vi "Martinas Aging Program v1.0a.vi"() -> ()   [LabVIEW 2011]
uses:
  SubVIs/Control 3.ctl
panel:
  in  "Scan Switch":T1=TRUE
  out "TIMER":dbl format="%<%H:%M:%S>t"
  in  "Delete from Menu Ring":bool
  in  "User Set?":bool
  out "Show me Scan \nSettings JV set":T2={"Light Intensity (Suns)"=1.0, "Stabilization Time (s)"=5.0, "Maximum Voltage (V)"=0.0, "Minimum Voltage (V)"=-1.0, "Range Options"=0, "Scan Direction\nDU (T), UD (F)"=TRUE, "Step Size (V)"=0.01, "Source Delay (s)"=0.15} {"Range Options" items=["Auto Range", "Semi-Auto Range", "100 uA", "1 mA", "10 mA", "100 mA", "1A"]}
  in  "Add to Menu ring":bool
  in  "Scan Setting Name":string
  in  "Scan Settings JV":T2={"Light Intensity (Suns)"=1.0, "Stabilization Time (s)"=5.0, "Maximum Voltage (V)"=0.0, "Minimum Voltage (V)"=-1.0, "Range Options"=0, "Scan Direction\nDU (T), UD (F)"=TRUE, "Step Size (V)"=0.01, "Source Delay (s)"=0.15} {"Range Options" items=["Auto Range", "Semi-Auto Range", "100 uA", "1 mA", "10 mA", "100 mA", "1A"]}
  in  "Scan settings":u16(ring) items=["Regular", "Inverted"]
  out "JV Curve":cluster{"Y":dbl[], "Y":dbl[]}[](graph)
  out "Table":string[][](table)
  in  "Logout":bool
  in  "Login":bool
  out "Username":string caption="Logged in as:"
  in  "Sort by":u16(ring) items=["Cell position", "Cell label", "Time in rig"]
  in  "Sort Queue":bool
  in  "Upload to the Queue":bool
  in  "Queue":T3(array[cluster])=[{"Measure?"=TRUE, "Area (cm^2)"=0.0, "Cell Label"="", "Cell Description"="", "Cell Position"=0, "Time in rig (h)"=0.0, "Time to next scan (min)"=0.0, "Scan number"=0.0, "When did you stick it in?"=0.0, "Time between scans (min)"=0.0, "Time of the last scan(min)"=0.0, "Scan settings in queue"=0}, {"Measure?"=TRUE, "Area (cm^2)"=0.0, "Cell Label"="", "Cell Description"="", "Cell Position"=0, "Time in rig (h)"=0.0, "Time to next scan (min)"=0.0, "Scan number"=0.0, "When did you stick it in?"=0.0, "Time between scans (min)"=0.0, "Time of the last scan(min)"=0.0, "Scan settings in queue"=0}, {"Measure?"=TRUE, "Area (cm^2)"=0.0, "Cell Label"="", "Cell Description"="", "Cell Position"=0, "Time in rig (h)"=0.0, "Time to next scan (min)"=0.0, "Scan number"=0.0, "When did you stick it in?"=0.0, "Time between scans (min)"=0.0, "Time of the last scan(min)"=0.0, "Scan settings in queue"=0}, {"Measure?"=TRUE, "Area (cm^2)"=0.0, "Cell Label"="", "Cell Description"="", "Cell Position"=0, "Time in rig (h)"=0.0, "Time to next scan (min)"=0.0, "Scan number"=0.0, "When did you stick it in?"=0.0, "Time between scans (min)"=0.0, "Time of the last scan(min)"=0.0, "Scan settings in queue"=0}, {"Measure?"=TRUE, "Area (cm^2)"=0.0, "Cell Label"="", "Cell Description"="", "Cell Position"=0, "Time in rig (h)"=0.0, "Time to next scan (min)"=0.0, "Scan number"=0.0, "When did you stick it in?"=0.0, "Time between scans (min)"=0.0, "Time of the last scan(min)"=0.0, "Scan settings in queue"=0}, {"Measure?"=TRUE, "Area (cm^2)"=0.0, "Cell Label"="", "Cell Description"="", "Cell Position"=0, "Time in rig (h)"=0.0, "Time to next scan (min)"=0.0, "Scan number"=0.0, "When did you stick it in?"=0.0, "Time between scans (min)"=0.0, "Time of the last scan(min)"=0.0, "Scan settings in queue"=0}, {"Measure?"=TRUE, "Area (cm^2)"=0.0, "Cell Label"="", "Cell Description"="", "Cell Position"=0, "Time in rig (h)"=0.0, "Time to next scan (min)"=0.0, "Scan number"=0.0, "When did you stick it in?"=0.0, "Time between scans (min)"=0.0, "Time of the last scan(min)"=0.0, "Scan settings in queue"=0}, {"Measure?"=TRUE, "Area (cm^2)"=0.0, "Cell Label"="", "Cell Description"="", "Cell Position"=0, "Time in rig (h)"=0.0, "Time to next scan (min)"=0.0, "Scan number"=0.0, "When did you stick it in?"=0.0, "Time between scans (min)"=0.0, "Time of the last scan(min)"=0.0, "Scan settings in queue"=0}, {"Measure?"=TRUE, "Area (cm^2)"=0.0, "Cell Label"="", "Cell Description"="", "Cell Position"=0, "Time in rig (h)"=0.0, "Time to next scan (min)"=0.0, "Scan number"=0.0, "When did you stick it in?"=0.0, "Time between scans (min)"=0.0, "Time of the last scan(min)"=0.0, "Scan settings in queue"=0}, {"Measure?"=TRUE, "Area (cm^2)"=0.0, "Cell Label"="", "Cell Description"="", "Cell Position"=0, "Time in rig (h)"=0.0, "Time to next scan (min)"=0.0, "Scan number"=0.0, "When did you stick it in?"=0.0, "Time between scans (min)"=0.0, "Time of the last scan(min)"=0.0, "Scan settings in queue"=0}, {"Measure?"=TRUE, "Area (cm^2)"=0.0, "Cell Label"="", "Cell Description"="", "Cell Position"=0, "Time in rig (h)"=0.0, "Time to next scan (min)"=0.0, "Scan number"=0.0, "When did you stick it in?"=0.0, "Time between scans (min)"=0.0, "Time of the last scan(min)"=0.0, "Scan settings in queue"=0}, {"Measure?"=TRUE, "Area (cm^2)"=0.0, "Cell Label"="", "Cell Description"="", "Cell Position"=0, "Time in rig (h)"=0.0, "Time to next scan (min)"=0.0, "Scan number"=0.0, "When did you stick it in?"=0.0, "Time between scans (min)"=0.0, "Time of the last scan(min)"=0.0, "Scan settings in queue"=0}, {"Measure?"=TRUE, "Area (cm^2)"=0.0, "Cell Label"="", "Cell Description"="", "Cell Position"=0, "Time in rig (h)"=0.0, "Time to next scan (min)"=0.0, "Scan number"=0.0, "When did you stick it in?"=0.0, "Time between scans (min)"=0.0, "Time of the last scan(min)"=0.0, "Scan settings in queue"=0}, {"Measure?"=TRUE, "Area (cm^2)"=0.0, "Cell Label"="", "Cell Description"="", "Cell Position"=0, "Time in rig (h)"=0.0, "Time to next scan (min)"=0.0, "Scan number"=0.0, "When did you stick it in?"=0.0, "Time between scans (min)"=0.0, "Time of the last scan(min)"=0.0, "Scan settings in queue"=0}, {"Measure?"=TRUE, "Area (cm^2)"=0.0, "Cell Label"="", "Cell Description"="", "Cell Position"=0, "Time in rig (h)"=0.0, "Time to next scan (min)"=0.0, "Scan number"=0.0, "When did you stick it in?"=0.0, "Time between scans (min)"=0.0, "Time of the last scan(min)"=0.0, "Scan settings in queue"=0}, {"Measure?"=TRUE, "Area (cm^2)"=0.0, "Cell Label"="", "Cell Description"="", "Cell Position"=0, "Time in rig (h)"=0.0, "Time to next scan (min)"=0.0, "Scan number"=0.0, "When did you stick it in?"=0.0, "Time between scans (min)"=0.0, "Time of the last scan(min)"=0.0, "Scan settings in queue"=0}] {"Scan settings in queue" items=["Regular", "Inverted"]; "Time of the last scan(min)" format="%<%H:%M:%S>t"; "When did you stick it in?" format="%<%H:%M:%S>t"; "Time to next scan (min)" format="%<%H:%M:%S>t"; "Time in rig (h)" format="%<%H:%M:%S>t"}
  in  "Save Spreadsheet Path":path
  in  "Save to Spreadsheet?":bool
  in  "Upload Spreadsheet path":path
  in  "Upload from Spreadsheet?":bool
  in  "stop":bool
  in  "Cell Settings Array":T4(array[cluster])=[{"Measure?"=TRUE, "Area (cm^2)"=0.0, "Cell Label"="", "Cell Description"="", "Time between scans (min)"=0.0, "Cell Position"=0, "Scan settings in queue"=0}, {"Measure?"=TRUE, "Area (cm^2)"=0.0, "Cell Label"="", "Cell Description"="", "Time between scans (min)"=0.0, "Cell Position"=0, "Scan settings in queue"=0}, {"Measure?"=TRUE, "Area (cm^2)"=0.0, "Cell Label"="", "Cell Description"="", "Time between scans (min)"=0.0, "Cell Position"=0, "Scan settings in queue"=0}, {"Measure?"=TRUE, "Area (cm^2)"=0.0, "Cell Label"="", "Cell Description"="", "Time between scans (min)"=0.0, "Cell Position"=0, "Scan settings in queue"=0}, {"Measure?"=TRUE, "Area (cm^2)"=0.0, "Cell Label"="", "Cell Description"="", "Time between scans (min)"=0.0, "Cell Position"=0, "Scan settings in queue"=0}, {"Measure?"=TRUE, "Area (cm^2)"=0.0, "Cell Label"="", "Cell Description"="", "Time between scans (min)"=0.0, "Cell Position"=0, "Scan settings in queue"=0}, {"Measure?"=TRUE, "Area (cm^2)"=0.0, "Cell Label"="", "Cell Description"="", "Time between scans (min)"=0.0, "Cell Position"=0, "Scan settings in queue"=0}, {"Measure?"=TRUE, "Area (cm^2)"=0.0, "Cell Label"="", "Cell Description"="", "Time between scans (min)"=0.0, "Cell Position"=0, "Scan settings in queue"=0}, {"Measure?"=TRUE, "Area (cm^2)"=0.0, "Cell Label"="", "Cell Description"="", "Time between scans (min)"=0.0, "Cell Position"=0, "Scan settings in queue"=0}, {"Measure?"=TRUE, "Area (cm^2)"=0.0, "Cell Label"="", "Cell Description"="", "Time between scans (min)"=0.0, "Cell Position"=0, "Scan settings in queue"=0}, {"Measure?"=TRUE, "Area (cm^2)"=0.0, "Cell Label"="", "Cell Description"="", "Time between scans (min)"=0.0, "Cell Position"=0, "Scan settings in queue"=0}, {"Measure?"=TRUE, "Area (cm^2)"=0.0, "Cell Label"="", "Cell Description"="", "Time between scans (min)"=0.0, "Cell Position"=0, "Scan settings in queue"=0}, {"Measure?"=TRUE, "Area (cm^2)"=0.0, "Cell Label"="", "Cell Description"="", "Time between scans (min)"=0.0, "Cell Position"=0, "Scan settings in queue"=0}, {"Measure?"=TRUE, "Area (cm^2)"=0.0, "Cell Label"="", "Cell Description"="", "Time between scans (min)"=0.0, "Cell Position"=0, "Scan settings in queue"=0}, {"Measure?"=TRUE, "Area (cm^2)"=0.0, "Cell Label"="", "Cell Description"="", "Time between scans (min)"=0.0, "Cell Position"=0, "Scan settings in queue"=0}, {"Measure?"=TRUE, "Area (cm^2)"=0.0, "Cell Label"="", "Cell Description"="", "Time between scans (min)"=0.0, "Cell Position"=0, "Scan settings in queue"=0}] {"Scan settings in queue" items=["Regular", "Inverted"]}
  # "Time between Scans (min)"
  # "On = working cell\nOff = not working cell"
  # "Area"
  # "Label"
  # "Comment"
  # "Cell position"
  # "Scan Settings"
  # "Time between Scans (min)"
  # "Time since the last scan (min)"
  # "Scan\nnumber"
  # "When did you stick it in?"
  # "Time of the last scan"
  # "On = working cell\nOff = not working cell"
  # "Area"
  # "Label"
  # "Comment"
  # "Cell position"
  # "Time in rig"
  # "Scan Settings"
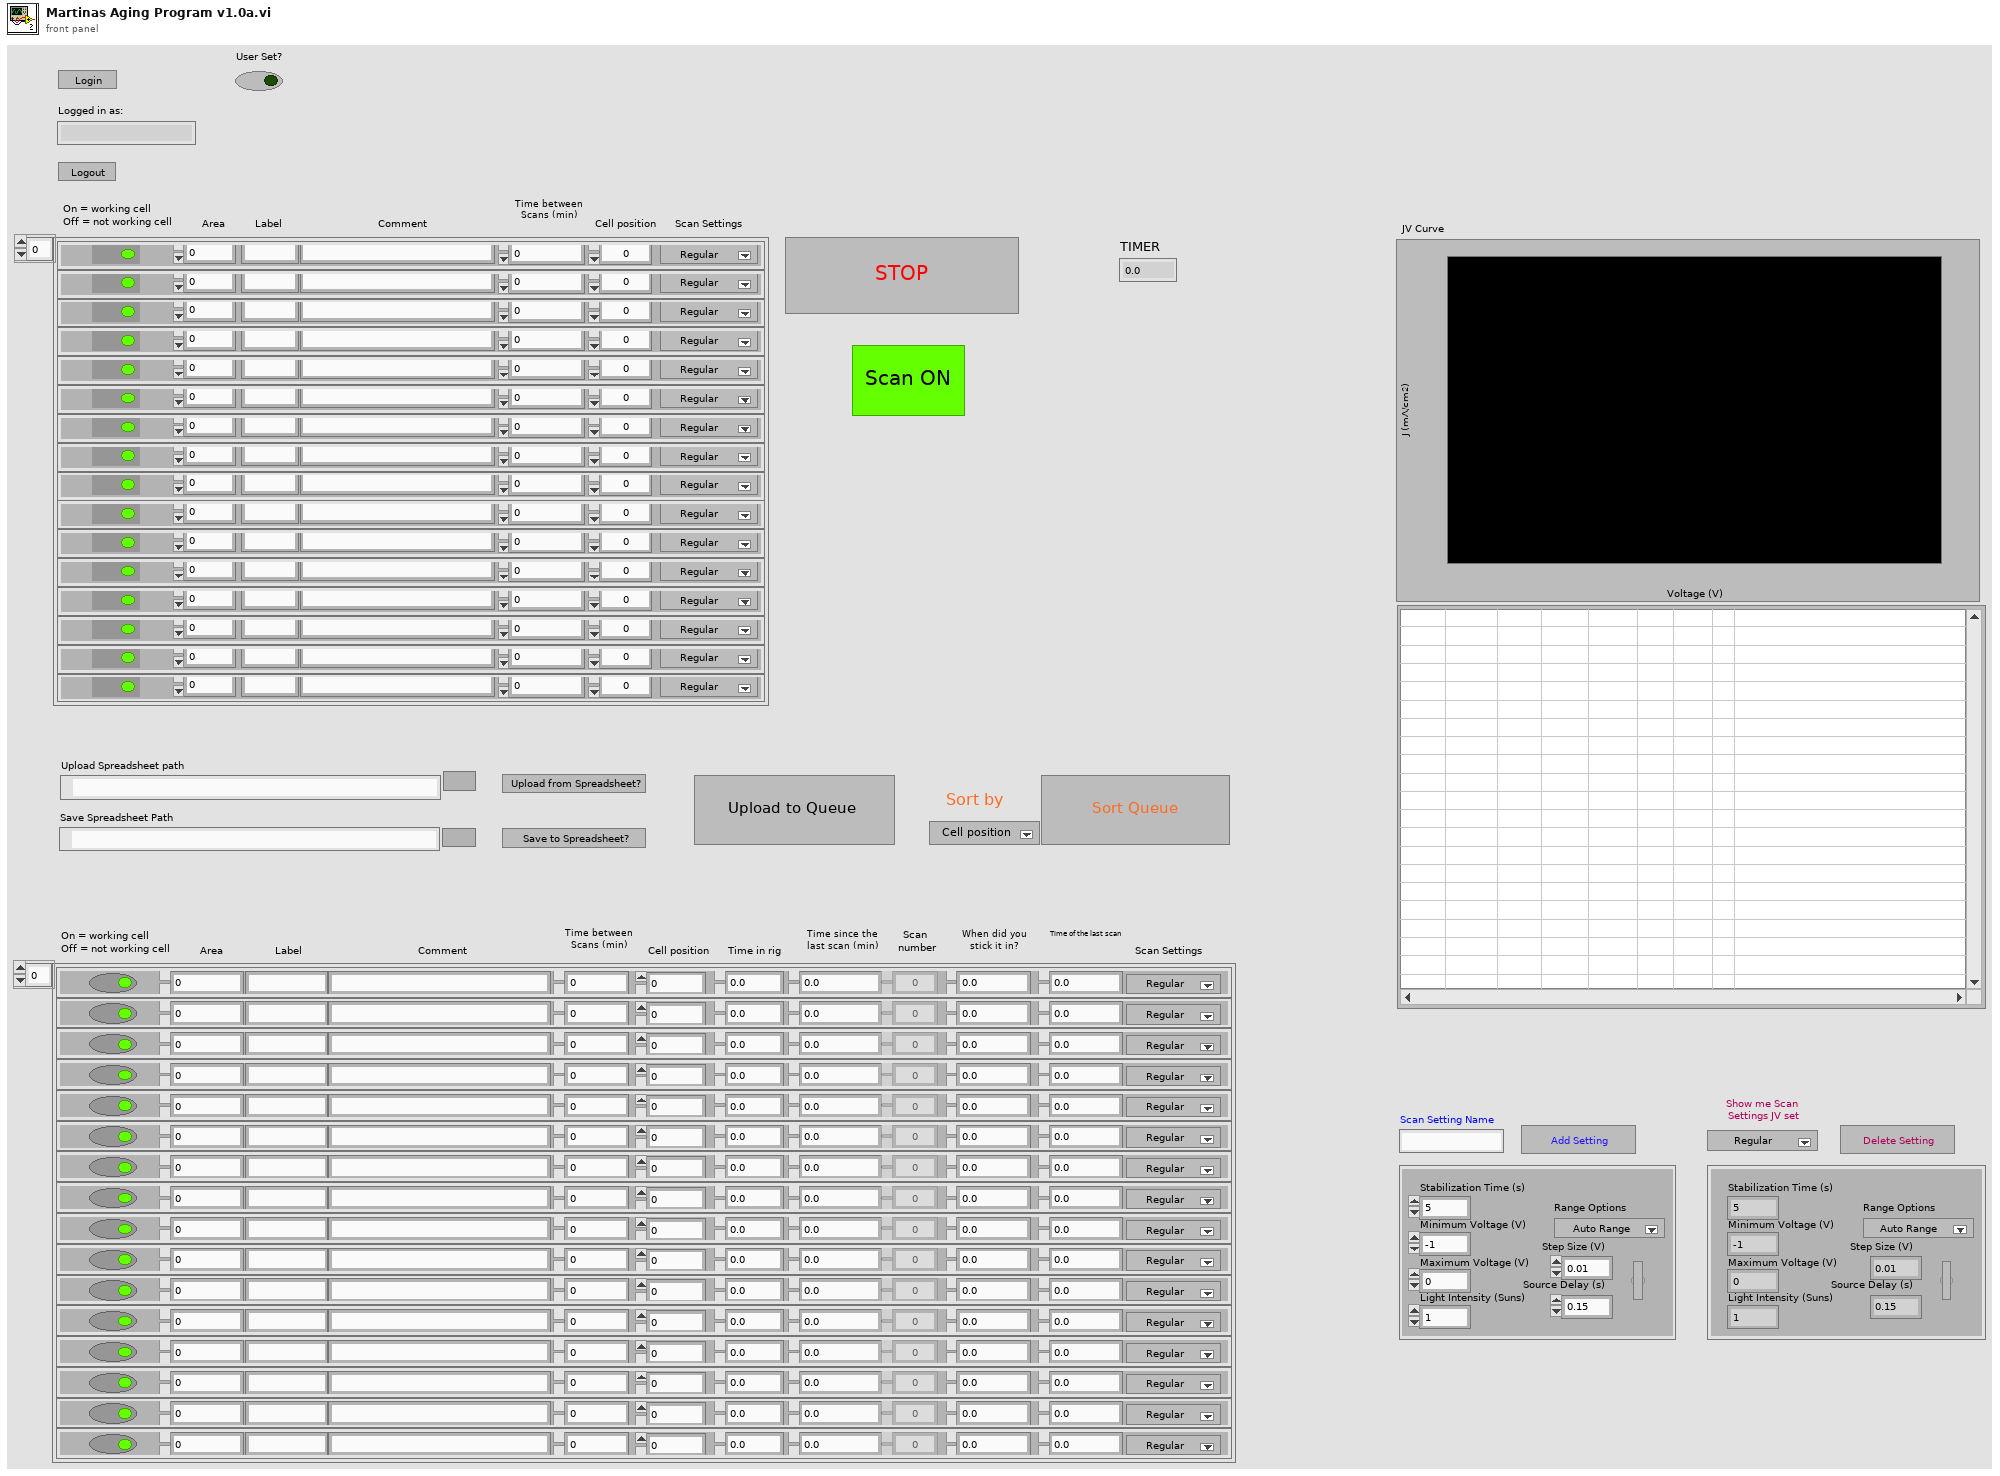
[diagram p1: front panel]
types:
  T1 = typedef "Control 3.ctl" = bool
  T2 = cluster{"Light Intensity (Suns)":dbl, "Stabilization Time (s)":dbl, "Maximum Voltage (V)":dbl, "Minimum Voltage (V)":dbl, "Range Options":u16, "Scan Direction\nDU (T), UD (F)":bool, "Step Size (V)":dbl, "Source Delay (s)":dbl}
  T3 = cluster{"Measure?":bool, "Area (cm^2)":dbl, "Cell Label":string, "Cell Description":string, "Cell Position":i32, "Time in rig (h)":dbl, "Time to next scan (min)":dbl, "Scan number":dbl, "When did you stick it in?":dbl, "Time between scans (min)":dbl, "Time of the last scan(min)":dbl, "Scan settings in queue":u16}[]
  T4 = cluster{"Measure?":bool, "Area (cm^2)":dbl, "Cell Label":string, "Cell Description":string, "Time between scans (min)":dbl, "Cell Position":i32, "Scan settings in queue":u16}[]
  T5 = cluster{"Light Intensity (Suns)":dbl, "Stabilization Time (s)":dbl, "Maximum Voltage (V)":dbl, "Minimum Voltage (V)":dbl, "Range Options":u16, "Scan Direction\nDU (T), UD (F)":bool, "Step Size (V)":dbl, "Source Delay (s)":dbl}[]
  T6 = enum8{"Enabled", "Disabled", "Disabled and Grayed Out"}
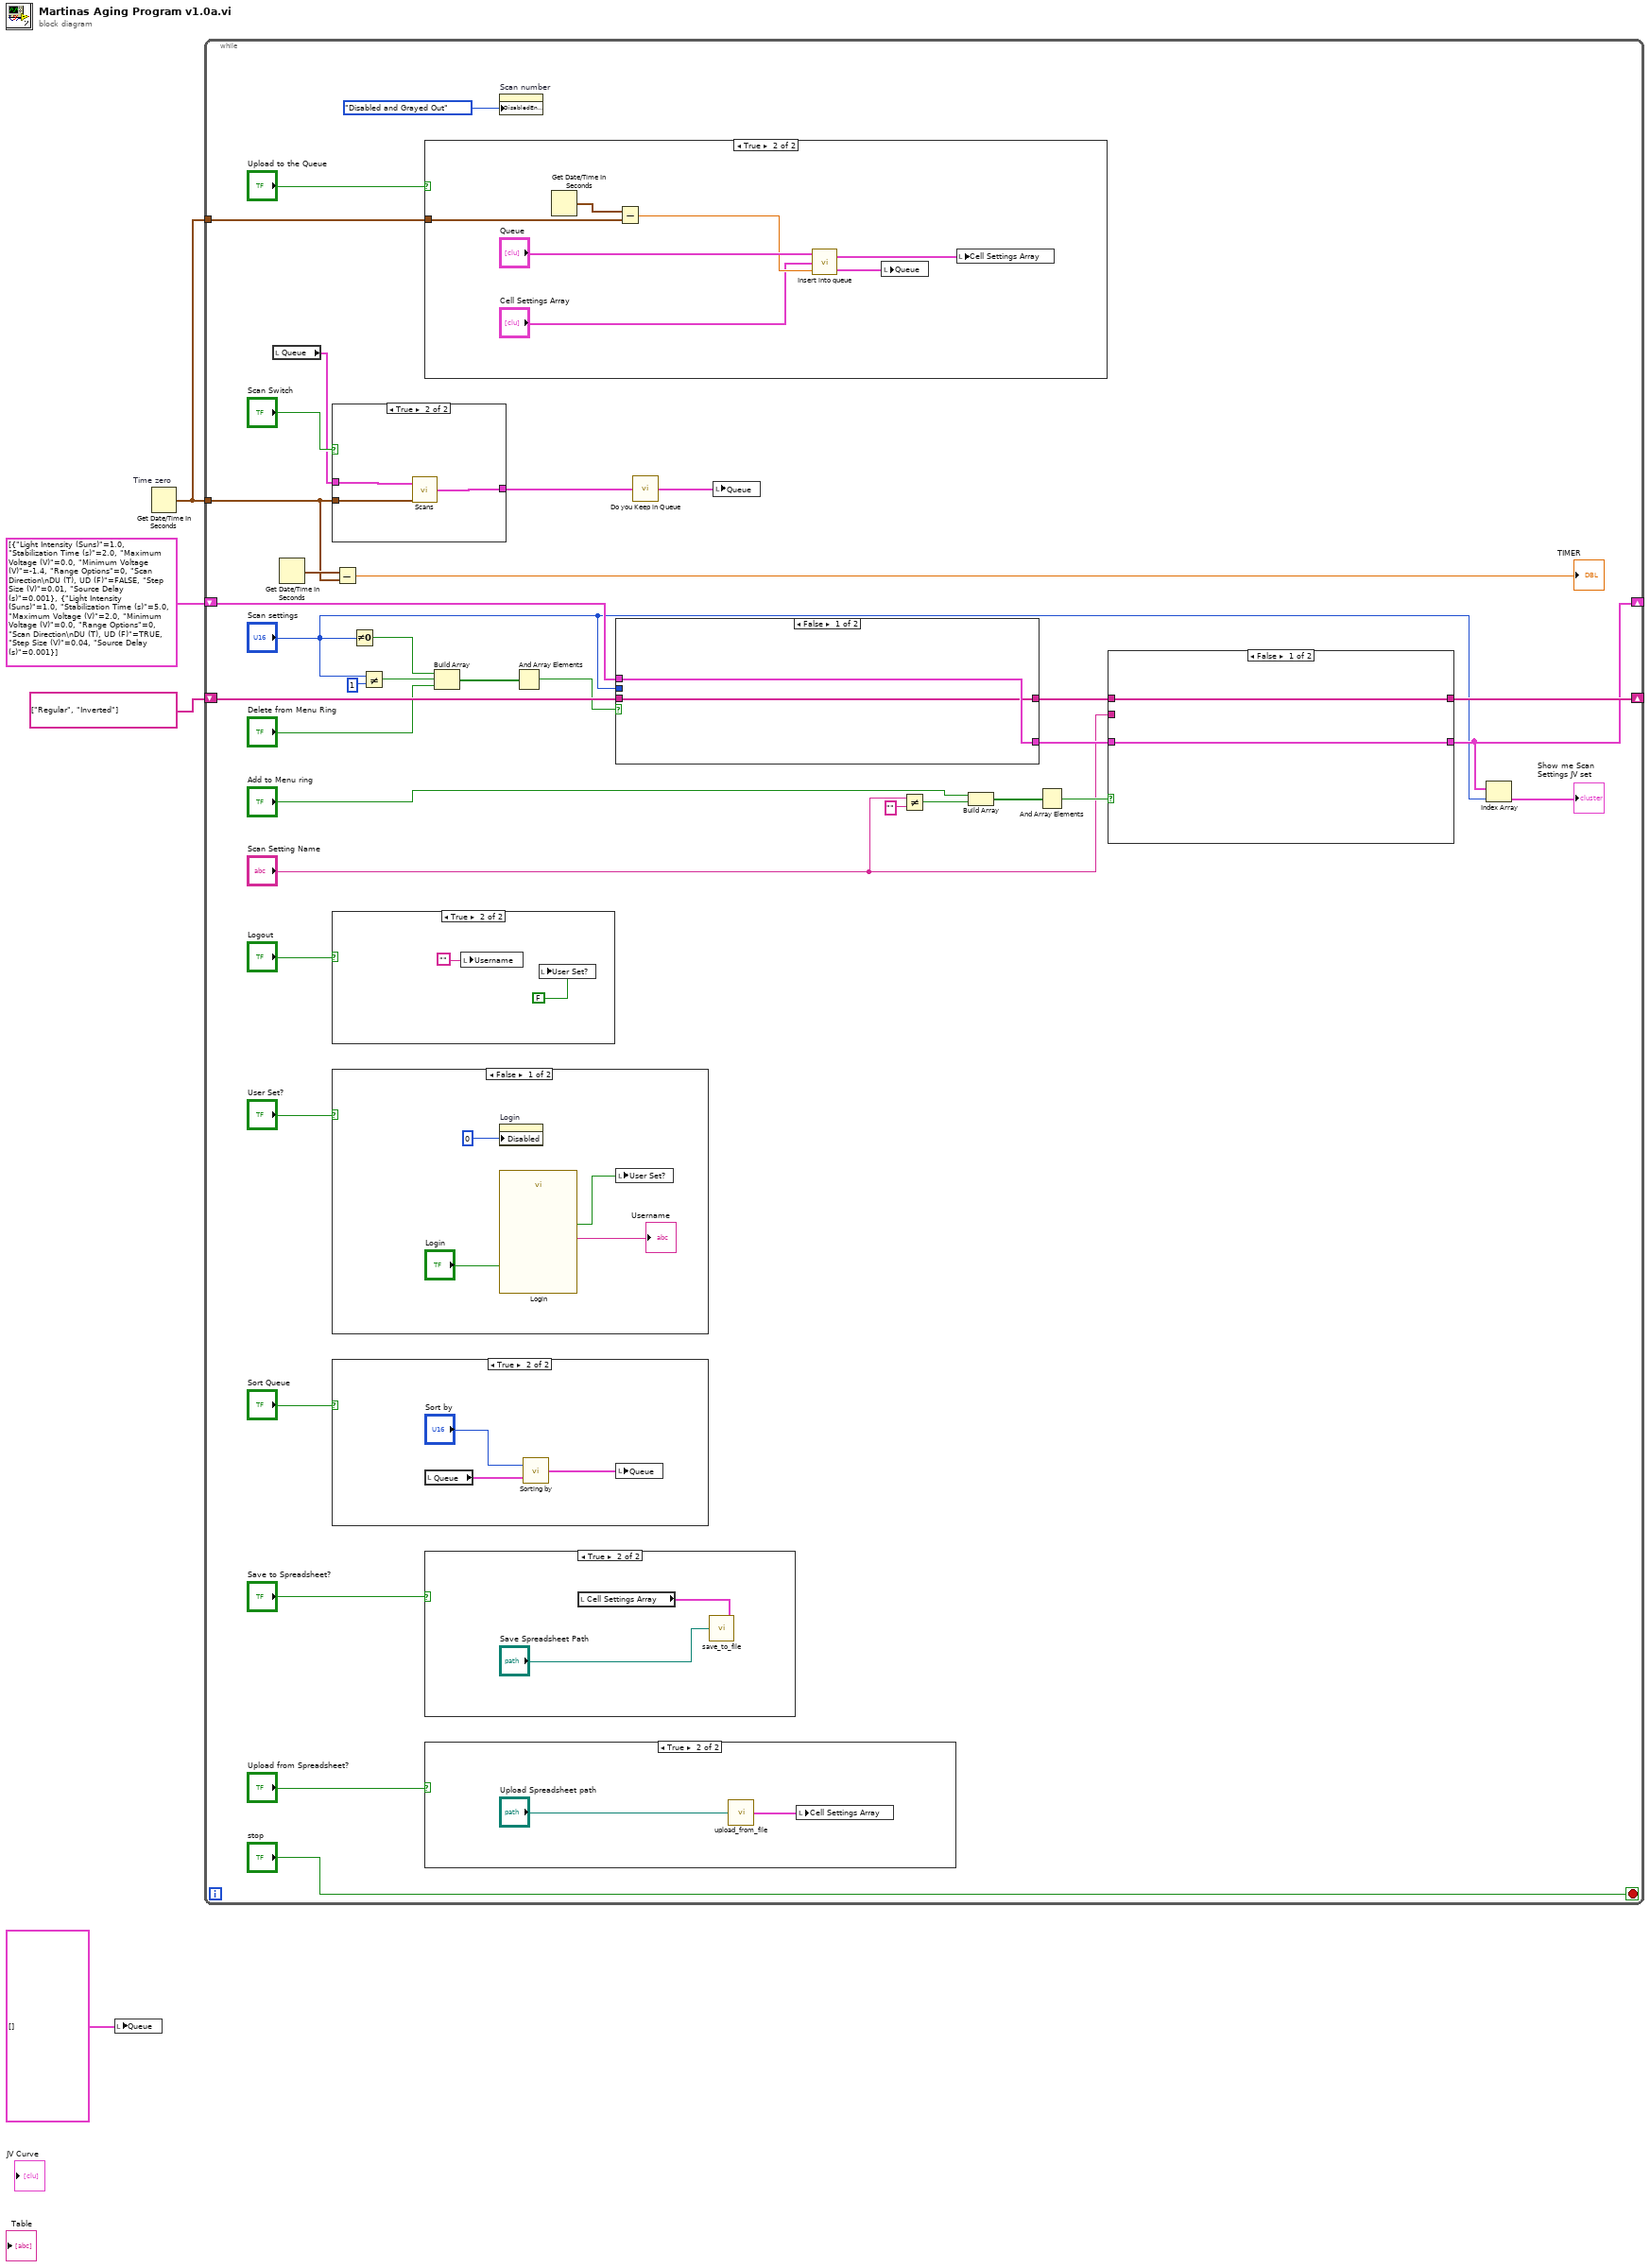
[diagram p0: block diagram]
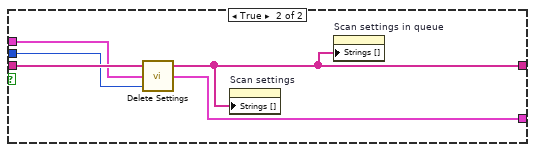
[diagram p3: hidden frame]
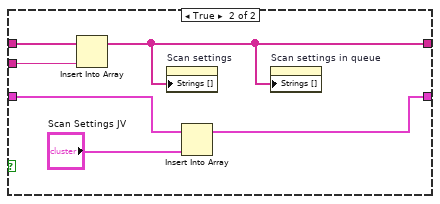
[diagram p4: hidden frame]
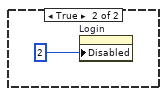
[diagram p6: hidden frame]
diagram:
  n1 = local write "Queue"(T3 [] ("Queue")) -> ()
  n2 = Get Date/Time In Seconds "Time zero"() -> (seconds since 1Jan1904=w1:timestamp)
  n3 = while {
    tunnel: w1 -> [w35]
    shift-right: [w30] -> _
    shift-left: T5 [{"Light Intensity (Suns)"=1.0, "Stabilization Time (s)"=2.0, "Maximum Voltage (V)"=0.0, "Minimum Voltage (V)"=-1.4, "Range Options"=0, "Scan Direction\nDU (T), UD (F)"=FALSE, "Step Size (V)"=0.01, "Source Delay (s)"=0.001}, {"Light Intensity (Suns)"=1.0, "Stabilization Time (s)"=5.0, "Maximum Voltage (V)"=2.0, "Minimum Voltage (V)"=0.0, "Range Options"=0, "Scan Direction\nDU (T), UD (F)"=TRUE, "Step Size (V)"=0.04, "Source Delay (s)"=0.001}] ("JV curve scan settings 2") -> [w27]
    shift-right: [w32] -> _
    shift-left: string[] ["Regular", "Inverted"] ("Strings []") -> [w28]
    tunnel: w1 -> [w7]
    stop <- "stop" stop-if-true
    n4 = local read "Queue"() -> (w5:T3)
    n5 = Get Date/Time In Seconds() -> (seconds since 1Jan1904=w9:timestamp)
    n6 = case shown="True" "Scan Switch" {
      tunnel: w5 -> [w41 w44]
      tunnel: w7 -> [_ w43]
      tunnel: [w41 w42] -> w8
      frame False {
      }
      frame True {
        n7 = call "Scans.vi"("Time zero (sec)"=w43, "Queue In"=w44) -> ("Queue"=w42:T3)
      }
    }
    n8 = case shown="True" "Logout" {
      frame False {
      }
      frame True {
        n9 = local write "Username"("") -> ()
        n10 = local write "User Set?"(FALSE) -> ()
      }
    }
    n11 = case shown="False" "User Set?" {
      frame False {
        n12 = property on="Login" class="Bool"("Disabled"=0) -> ()  [unwired: 2 in, 2 out]
        n13 = call "Login"("Enable"="Login") -> ("Username"=→"Username":string, "OK"=w62:bool)  [unwired: 16 in, 1 out]
        n14 = local write "User Set?"(w62) -> ()
      }
      frame True {
        n15 = property on="Login" class="Bool"("Disabled"=2) -> ()  [unwired: 2 in, 2 out]
      }
    }
    n16 = case shown="True" "Sort Queue" {
      frame False {
      }
      frame True {
        n17 = local read "Queue"() -> (w68:T3)
        n18 = call "Sorting by.vi"("Queue"=w68, "Sort by"="Sort by") -> ("Queue 2"=w67:T3)
        n19 = local write "Queue"(w67) -> ()
      }
    }
    n20 = Subtract(x=w9, y=w7) -> (x-y=→"TIMER":dbl)
    n21 = Not Equal To 0?(x="Scan settings") -> (x != 0?=w24:bool)
    n22 = Not Equal?(x="Scan settings", y=u16 1) -> (x != y?=w21:bool)
    n23 = case shown="True" "Upload to the Queue" {
      tunnel: w35 -> [_ w76]
      frame False {
      }
      frame True {
        n24 = Get Date/Time In Seconds() -> (seconds since 1Jan1904=w75:timestamp)
        n25 = Subtract(x=w75, y=w76) -> (x-y=w73:dbl)
        n26 = call "Insert into queue.vi"("When did you stick it in?"=w73, "Cell Settings Array"="Cell Settings Array", "Queue In"="Queue") -> ("Queue"=w71:T3, "Cell Settings Array 2"=w70:T4)
        n27 = local write "Queue"(w71) -> ()
        n28 = local write "Cell Settings Array"(w70) -> ()
      }
    }
    n29 = case shown="True" "Save to Spreadsheet?" {
      frame False {
      }
      frame True {
        n30 = local read "Cell Settings Array"() -> (w77:T4)
        n31 = call "save_to_file.vi"("Cell Settings Array 2"=w77, "Save Path"="Save Spreadsheet Path") -> ()
      }
    }
    n32 = case shown="True" "Upload from Spreadsheet?" {
      frame False {
      }
      frame True {
        n33 = call "upload_from_file.vi"("Spreadsheet path"="Upload Spreadsheet path") -> ("Cell Settings Array"=w79:T4)
        n34 = local write "Cell Settings Array"(w79) -> ()
      }
    }
    n35 = Build Array(w24, w21, "Delete from Menu Ring") -> (w19:bool[])
    n36 = property on="Scan number" class="DigNum (strict)"("DisabledEnum"=T6."Disabled and Grayed Out" ("Disabled")) -> ()  [unwired: 2 in, 2 out]
    n37 = And Array Elements(Boolean array=w19) -> (logical AND=w18:bool)
    n38 = case shown="False" w18 {
      tunnel: w28 -> [w45 w51]
      tunnel: w27 -> [w46 w50]
      tunnel: "Scan settings" -> [_ w49]
      tunnel: [w45 w48] -> w26
      tunnel: [w46 w47] -> w25
      frame False {
      }
      frame True {
        n39 = call "Delete Settings.vi"("Scan settings"=w49, "JV curve scan settings"=w50, "Strings In"=w51) -> ("JV curve scan settings Out"=w47:T5, "Strings Out"=w48:string[])  [unwired: 1 out]
        n40 = property on="Scan settings" class="Ring (strict)"("Strings []"=w48) -> ()  [unwired: 2 in, 2 out]
        n41 = property on="Scan settings in queue" class="Ring (strict)"("Strings []"=w48) -> ()  [unwired: 2 in, 2 out]
      }
    }
    n42 = call "Do you Keep in Queue.vi"("Queue In"=w8) -> ("queue Out"=w10:T3)
    n43 = local write "Queue"(w10) -> ()
    n44 = Not Equal?(x="Scan Setting Name", y="") -> (x != y?=w15:bool)
    n45 = Build Array("Add to Menu ring", w15) -> (w16:bool[])
    n46 = And Array Elements(Boolean array=w16) -> (logical AND=w13:bool)
    n47 = case shown="False" w13 {
      tunnel: w25 -> [w53 w59]
      tunnel: [w53 w58] -> w30
      tunnel: w26 -> [w52 w55]
      tunnel: [w52 w56] -> w32
      tunnel: "Scan Setting Name" -> [_ w54]
      frame False {
      }
      frame True {
        n48 = Insert Into Array(array=w55, new element=w54) -> (w56:string[])  [unwired: 1 in]
        n49 = property on="Scan settings" class="Ring (strict)"("Strings []"=w56) -> ()  [unwired: 2 in, 2 out]
        n50 = Insert Into Array(array=w59, new element="Scan Settings JV") -> (w58:T5)  [unwired: 1 in]
        n51 = property on="Scan settings in queue" class="Ring (strict)"("Strings []"=w56) -> ()  [unwired: 2 in, 2 out]
      }
    }
    n52 = Index Array(array=w30, index="Scan settings") -> (element=→"Show me Scan \nSettings JV set":T2)
  }
